vi "WriteData.vi"(8 "Error In":errorcluster, 10 "Data":string, 11 "object in":refnum<class "DataSource.lvclass">) -> (0 "Error Out":errorcluster, 3 "object out":refnum<class "DataSource.lvclass">)   [LabVIEW 2020, in "DataSource.lvclass"]
uses:
  DataSource.lvclass
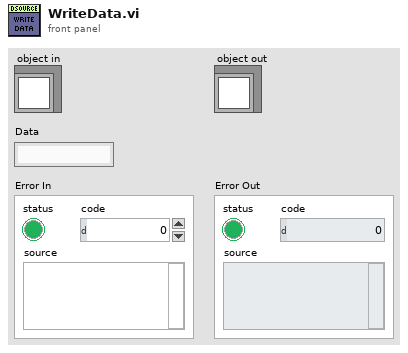
[diagram p1: front panel]
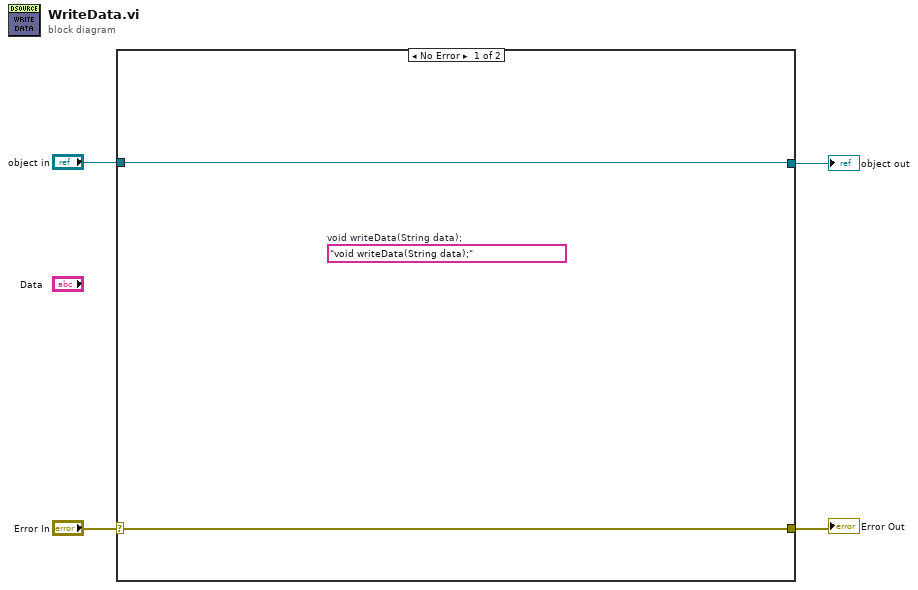
[diagram p0: block diagram]
diagram:
  n1 = case shown="No Error" "Error In" {
    selector: "Error In" -> [w6 w8]
    tunnel: [w6 w8] -> w3
    tunnel: [w5 w7] -> w1
    tunnel: "object in" -> [w5 w7]
    frame No Error {
      (unwired) "void writeData(String data);"  # void writeData(String data);
    }
    frame Error {
    }
  }
  "Error Out" <- w3
  "object out" <- w1
